vi "Launch Feature Test View.vi"(8 "error in (no error)":errorcluster, 11 "Example Controller Actor in":refnum<class "Example Controller Actor.lvclass">) -> (0 "error out":errorcluster, 3 "Example Controller Actor out":refnum<class "Example Controller Actor.lvclass">)   [LabVIEW 2023, in "Example Event Actors.lvlib" / "Example Controller Actor.lvlib" / "Example Controller Actor.lvclass"]
uses:
  Example Controller Actor.lvclass
  Example View Actor/Example View Actor 2/Example View Actor 2.lvclass
  View Actor/View Actor.lvclass/View Actor.ctl
  View Actor/properties/Write Name.vi
  Controller Actor/Controller Actor.lvclass
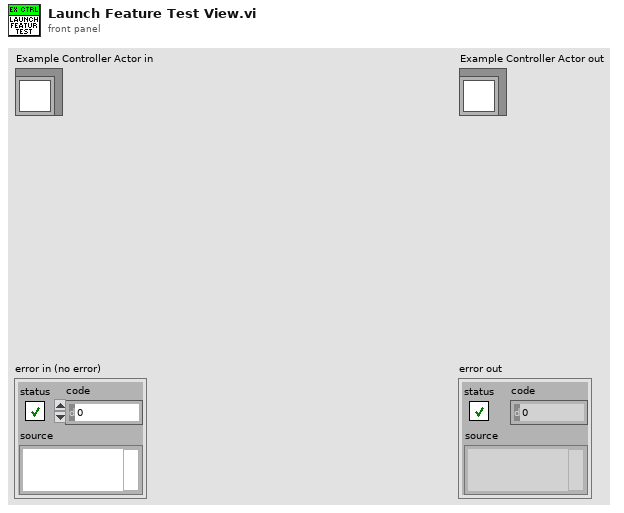
[diagram p1: front panel]
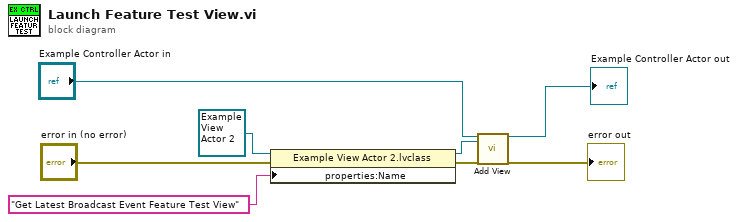
[diagram p0: block diagram]
diagram:
  n1 = property class="Example View Actor 2.lvclass"(reference=refnum<class "Example View Actor 2.lvclass"> refnum ("Example View Actor 2.lvlib:Example View Actor 2.lvclass"), error in="error in (no error)", "properties:Name"="Get Latest Broadcast Event Feature Test View" ("Debug Alias")) -> (reference out=w7:refnum<class "Example View Actor 2.lvclass">, error out=w6:errorcluster)
  n2 = call "Add View.vi"("Controller Actor in"="Example Controller Actor in", "View Actor"=w7, "error in (no error)"=w6) -> ("Controller Actor out"=→"Example Controller Actor out":refnum<class "Example Controller Actor.lvclass">, "error out"=→"error out":errorcluster)  [unwired: 14 in, 1 out]
